vi "Handle NVM.vi"(0 "Stand in":refnum<class "Stand.lvclass">, 11 "error in (no error)":errorcluster) -> (4 "Stand out":refnum<class "Stand.lvclass">, 15 "error out":errorcluster)   [LabVIEW 2019, in "Stand.lvclass"]
uses:
  Stand.lvclass
  Stand.lvclass/Stand.ctl
  Sig_AI_class/Sig_AI.lvclass/Sig_AI.ctl
  AnalogComparator_class/AnalogComparator.lvclass/AnalogComparator.ctl
  AnalogComparator_class/GetStatus.vi
  AnalogComparator_class/GetTh.vi
  ValveModbus_class/ValveModbus.lvclass
  Sig_AI_class/Sig_AI.lvclass
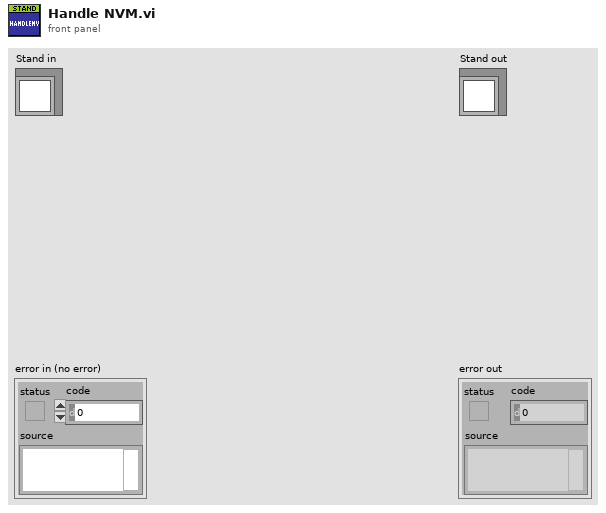
[diagram p1: front panel]
types:
  T1 = typedef "AI_Data.ctl" = cluster{"Raw":dbl, "Scaled":dbl, "OutOfRangeMax":bool, "OutOfRangeMin":bool, "HIHI":bool, "HI":bool, "LO":bool, "LOLO":bool, "OutOfRangeMax_val":dbl, "OutOfRangeMin_val":dbl, "HIHI_val":dbl, "HI_val":dbl, "LO_val":dbl, "LOLO_val":dbl}
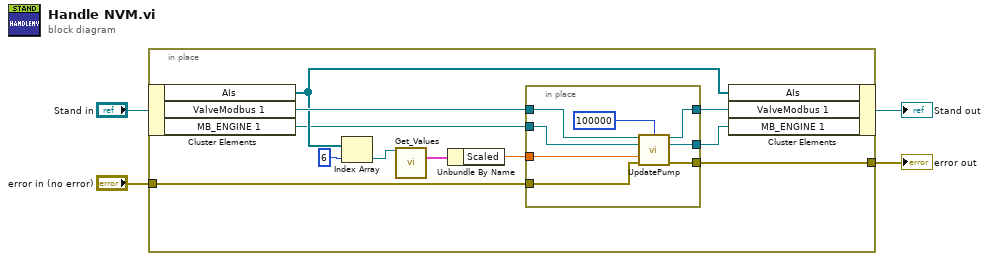
[diagram p0: block diagram]
diagram:
  n1 = in-place {
    in-place-border: "error in (no error)" -> [w13]
    in-place-border: [w12] -> w2
    n2 = in-place-cluster #1("Stand in") -> ("AIs"=w11:refnum<class "Sig_AI.lvclass">[], "ValveModbus 1"=w15:refnum<class "ValveModbus.lvclass">, "MB_ENGINE 1"=w6:refnum<class "MB_ENGINE.lvclass">)
    n3 = Index Array(array=w11, index=6) -> (element=w9:refnum<class "Sig_AI.lvclass">)
    n4 = call "Get_Values.vi"("reference in"=w9) -> ("Data"=w8:T1)  [unwired: 13 in, 1 out]
    n5 = Unbundle By Name(w8) -> ("Scaled"=w7:dbl)
    n6 = in-place {
      in-place-border: w15 -> [w22]
      in-place-border: [w21] -> w14
      in-place-border: w13 -> [w20]
      in-place-border: [w19] -> w12
      in-place-border: w7 -> [w18]
      in-place-border: w6 -> [w17]
      in-place-border: [w16] -> w5
      n7 = call "UpdatePump.vi"("Pump_1AI_1DO_2DI in"=w22, "ARG U32"=100000, "MB_ENGINE"=w17, "pressur"=w18, "error in (no error)"=w20) -> ("Pump_1AI_1DO_2DI out"=w21:refnum<class "ValveModbus.lvclass">, "class data out"=w16:refnum<class "MB_ENGINE.lvclass">, "error out"=w19:errorcluster)  [unwired: 8 in]
    }
    n8 = in-place-cluster #1("AIs"=w11, "ValveModbus 1"=w14, "MB_ENGINE 1"=w5) -> (→"Stand out":refnum<class "Stand.lvclass">)
  }
  "error out" <- w2
